vi "format output.vi"(8 "error in (no error)":errorcluster, 9 "Search for String":string, 10 "Regular Expression":string, 11 "Input String":string) -> (0 "error out":errorcluster, 3 "Output":dbl)   [LabVIEW 2017, in "MicrowaveAmplifier.lvlib"]
uses:
  MicrowaveAmplifier.lvlib
  <vilib>/regexp/Match Regular Expression.xnode
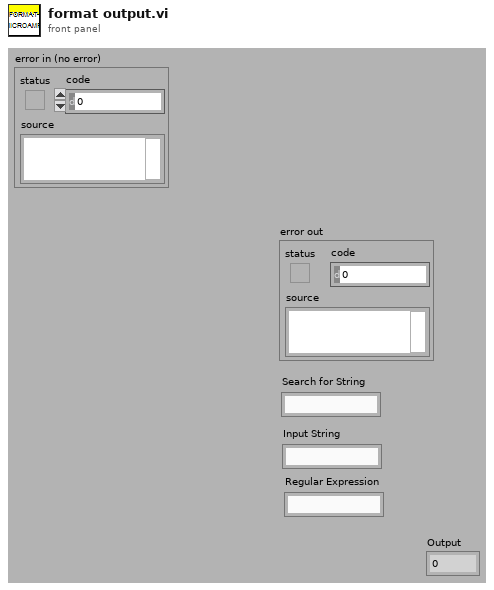
[diagram p1: front panel]
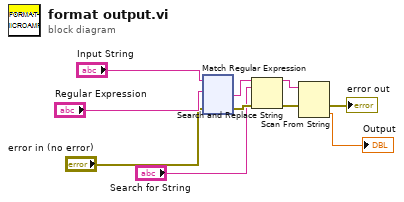
[diagram p0: block diagram]
diagram:
  n1 = xnode "Match Regular Expression"("input string"="Input String", "regular expression"="Regular Expression", "error in"="error in (no error)") -> ("after match"=w10:string, "error out"=w8:errorcluster)  [unwired: 3 in, 3 out]
  n2 = Search and Replace String(input string=w10, search string="Search for String", error in=w8) -> (result string=w9:string, error out=w7:errorcluster)  [unwired: 5 in, 2 out]
  n3 = Scan From String(input string=w9, error in=w7) -> (error out=→"error out":errorcluster, output 1=→"Output":dbl)  [unwired: 3 in, 2 out]
